vi "Temp Control--SubVI.vi"(4 "Instance":i32=1, 6 "Temp Control in":bool, 8 "error in":errorcluster, 9 "Control Mode (Auto)":u16(ring)=10 items=["Off"=62, "Auto"=10, "Manual"=54], 10 "Get/Set":enum16{"Get", "Set"}(ring), 11 "Watlow F4T in":refnum<class "Watlow F4T.lvclass">) -> (0 "error out":errorcluster, 2 "Temp Control":bool, 3 "Watlow F4T out":refnum<class "Watlow F4T.lvclass">)   [LabVIEW 2024, in "Watlow F4T.lvclass"]
uses:
  Watlow F4T.lvclass
  Private/Controls/Standard Bus Commands--Enum.ctl
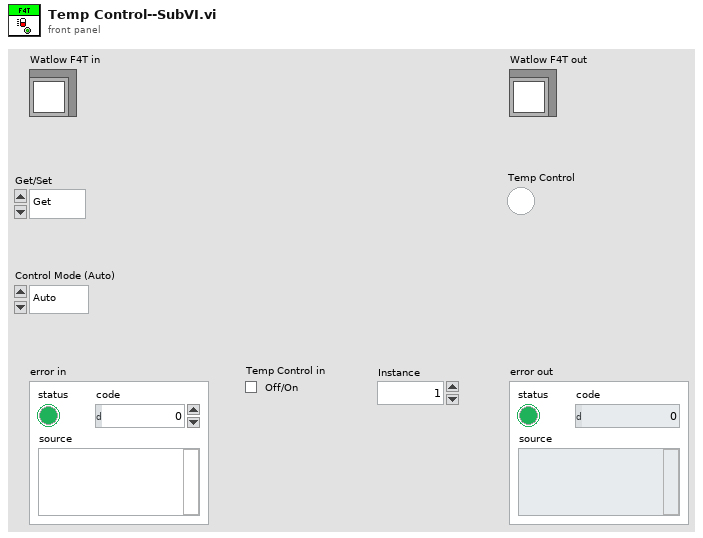
[diagram p1: front panel]
types:
  T1 = typedef "Watlow F4T.lvclass/Standard Bus Commands--Enum.ctl" = enum16{"Remote Setpoint", "Remote Mode", "Temp Feedback", "Target Setpoint", "Current Setpoint", "Setpoint Lower Limit", "Setpoint Upper Limit", "Ramp Rate Y", "Ramp Rate X", "Ramp Rate Action", "Temp Control State", "Temp Control Mode", "Power", "Heat Power", "Cool Power"}
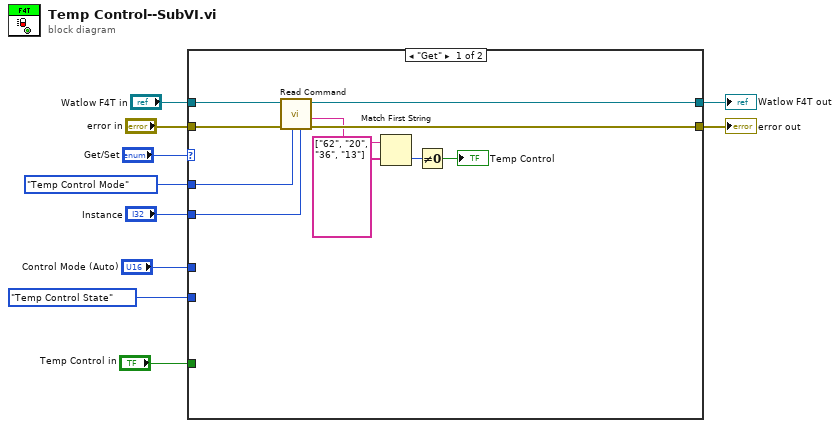
[diagram p0: block diagram]
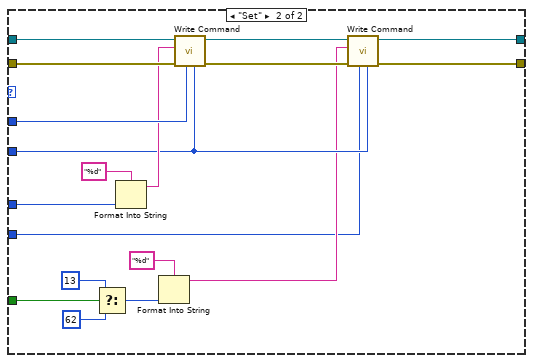
[diagram p2: hidden frame]
diagram:
  n1 = case shown="\"Get\"" "Get/Set" {
    tunnel: "Watlow F4T in" -> [w20 w38]
    tunnel: [w19 w31] -> w9
    tunnel: "error in" -> [w18 w37]
    tunnel: [w17 w30] -> w7
    tunnel: Standard_Bus_Commands--Enum."Temp Control Mode" ("Commands") -> [w16 w36]
    tunnel: "Instance" -> [w15 w29]
    tunnel: "Temp Control in" -> [_ w26]
    tunnel: "Control Mode (Auto)" -> [_ w22]
    tunnel: Standard_Bus_Commands--Enum."Temp Control State" ("Commands") -> [_ w21]
    frame "Get" {
      n2 = call "Read Command.vi"("Instance"=w15, "Commands"=w16, "error in (no error)"=w18, "Watlow F4T In"=w20) -> ("error out"=w17:errorcluster, "Value Out"=w12:string, "Watlow F4T out"=w19:refnum<class "Watlow F4T.lvclass">)  [unwired: 5 in]
      n3 = Match First String(2:string[] ["62", "20", "36", "13"] ("string array"), 3:w12) -> (0:w13:i32)  [unwired: 1 out]
      n4 = Not Equal To 0?(x=w13) -> (x != 0?=→"Temp Control":bool)
    }
    frame "Set" {
      n5 = Select(t=13, s=w26, f=62) -> (s? t:f=w25:i32)
      n6 = Format Into String(format string="%d", w22) -> (resulting string=w34:string)  [unwired: 2 in, 1 out]
      n7 = Format Into String(format string="%d", w25) -> (resulting string=w23:string)  [unwired: 2 in, 1 out]
      n8 = call "Write Command.vi"("Instance"=w29, "Commands"=w36, "error in (no error)"=w37, "Set Value"=w34, "Watlow F4T In"=w38) -> ("error out"=w33:errorcluster, "Watlow F4T out"=w32:refnum<class "Watlow F4T.lvclass">)  [unwired: 5 in]
      n9 = call "Write Command.vi"("Instance"=w29, "Commands"=w21, "error in (no error)"=w33, "Set Value"=w23, "Watlow F4T In"=w32) -> ("error out"=w30:errorcluster, "Watlow F4T out"=w31:refnum<class "Watlow F4T.lvclass">)  [unwired: 5 in]
    }
  }
  "Watlow F4T out" <- w9
  "error out" <- w7
